vi "Execute.vi"(8 "error in (no error)":errorcluster, 9 "Consumer Queues in":T1, 10 "UI Process Command in":refnum<class "Stop UI Process.lvclass">, 11 "UI Process Data in":T2) -> (0 "error out":errorcluster, 1 "Consumer Queues out":T1, 2 "Stop?":bool, 3 "UI Process Data out":T2)   [LabVIEW 2019, in "User Interface Process.lvlib" / "Stop UI Process.lvclass"]
uses:
  Stop UI Process.lvclass
  UI Process Data.ctl
  TS Framework/ExeLogging/UI Logger/UI Logger.lvclass
  UI State.ctl
  TS Framework/Consumer Queues.ctl
  Generic UI Command/Generic UI Process Command.lvclass
  DAC Process/Generic DAC Command/Generic DAC Process Command.lvclass
  Trig Process/Generic Trig Command/Generic Trig Process Command.lvclass
  User Interface Process.lvlib
  TS Framework/TS Framework.lvlib
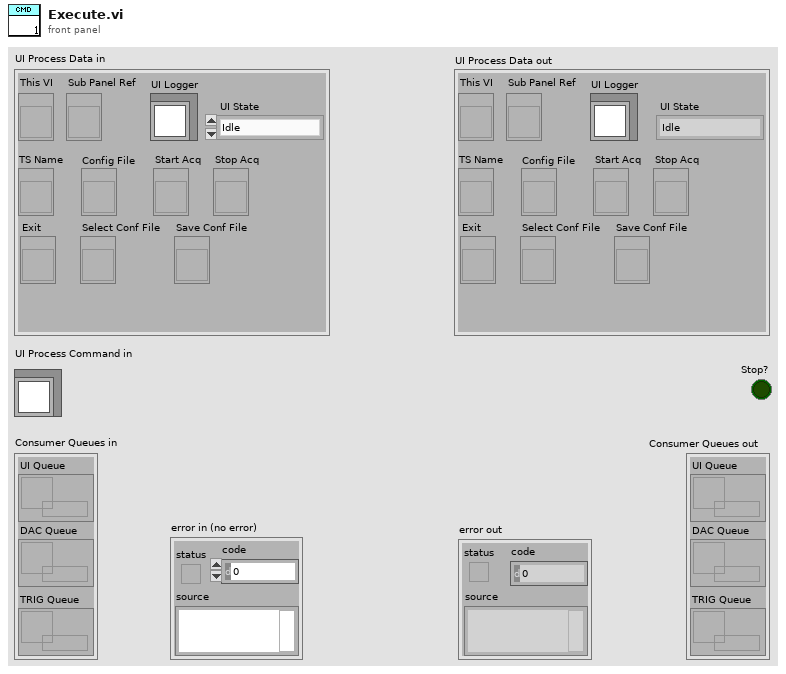
[diagram p1: front panel]
types:
  T1 = typedef "TS Framework.lvlib/Consumer Queues.ctl" = cluster{"UI Queue":refnum<queue>, "DAC Queue":refnum<queue>, "TRIG Queue":refnum<queue>}
  T2 = typedef "User Interface Process.lvlib/UI Process Data.ctl" = cluster{"This VI":refnum<vi>, "Sub Panel Ref":refnum<vi>, "UI Logger":refnum<class "UI Logger.lvclass">, "TS Name":refnum<vi>, "Config File":refnum<vi>, "Start Acq":refnum<vi>, "Stop Acq":refnum<vi>, "Exit":refnum<vi>, "Select Conf File":refnum<vi>, "Save Conf File":refnum<vi>, "UI State":T3}
  T3 = typedef "User Interface Process.lvlib/UI State.ctl" = enum16{"Idle", "Acquiring"}
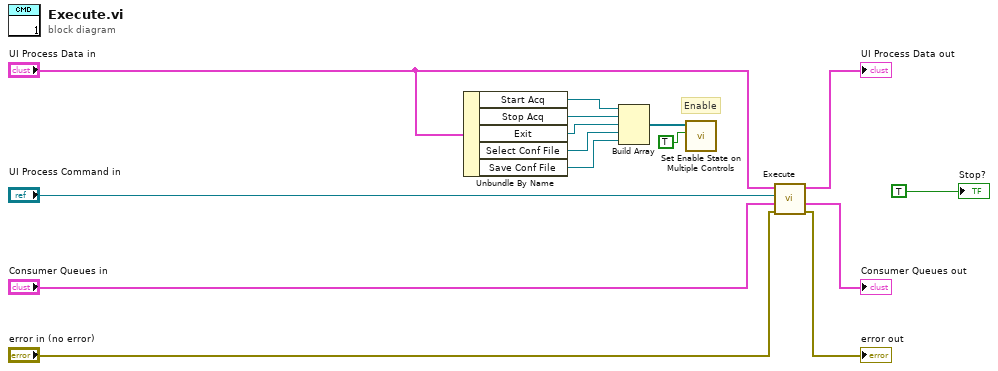
[diagram p0: block diagram]
diagram:
  # "Enable"
  n1 = Unbundle By Name("UI Process Data in") -> ("Start Acq"=w12:refnum<vi>, "Stop Acq"=w11:refnum<vi>, "Exit"=w10:refnum<vi>, "Select Conf File"=w9:refnum<vi>, "Save Conf File"=w8:refnum<vi>)
  n2 = Build Array(w12, w11, w10, w9, w8) -> (w13:refnum<vi>[])
  n3 = call "Set Enable State on Multiple Controls.vi"("Enable?"=TRUE, "Controls"=w13) -> ()  [unwired: 10 in]
  n4 = call-parent "Execute.vi"("error in (no error)"="error in (no error)", "Consumer Queues in"="Consumer Queues in", "UI Process Command in"="UI Process Command in", "UI Process Data in"="UI Process Data in") -> ("error out"=→"error out":errorcluster, "Consumer Queues out"=→"Consumer Queues out":T1, "UI Process Data out"=→"UI Process Data out":T2)  [unwired: 4 in, 1 out]
  "Stop?" <- TRUE
